vi "Serial.FrameCapture.vi"(7 "Over Time(mS)":u32=3000, 8 "error in (no error)":errorcluster caption="错误输入（无错误）", 9 "Input Text":string, 10 "baud rate (9600)":u32=9600 caption="BateRate(9600)", 11 "Serial":refnum<visa-resource-name>) -> (0 "error out":errorcluster caption="错误输出", 1 "Capture Text":string, 3 "Find?":bool)   [LabVIEW 2012, in "Lib_UEL.ATE.lvlib" / "Lib_2Voice.lvlib"]
uses:
  Lib_2Voice.lvlib
  <vilib>/Instr/_visa.llb/VISA Configure Serial Port (Instr).vi
panel:
  out "替换后偏移量":i32
  out "Time Count":u32
  in  "停止":bool
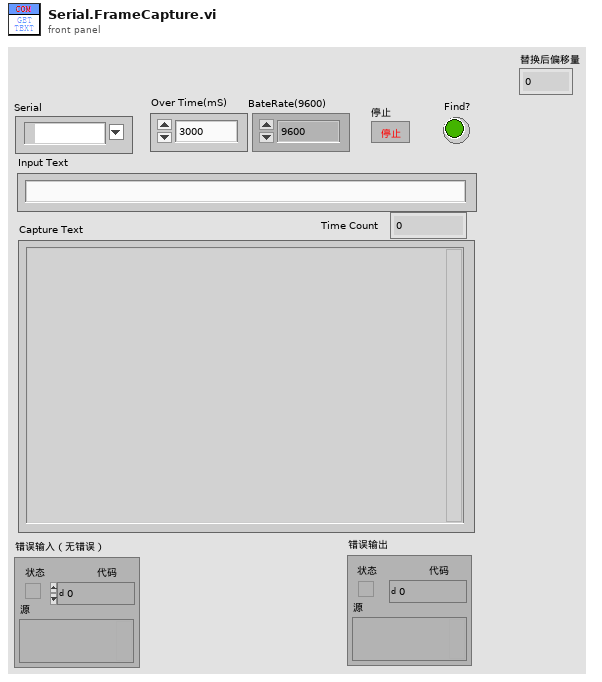
[diagram p1: front panel]
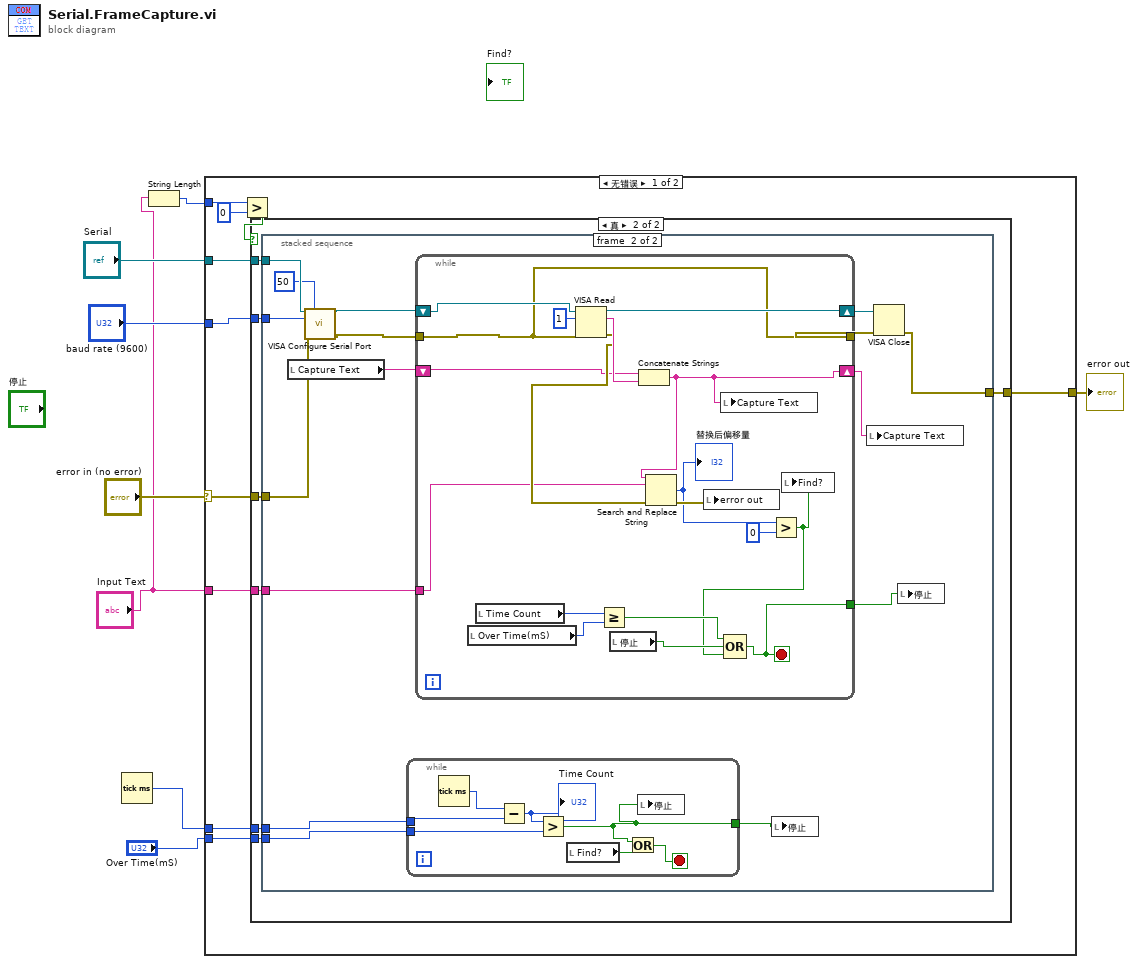
[diagram p0: block diagram]
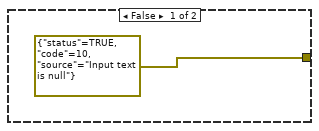
[diagram p2: hidden frame]
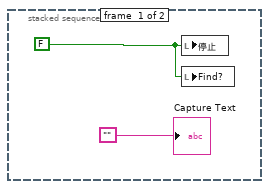
[diagram p3: hidden frame]
diagram:
  n1 = Tick Count (ms)() -> (millisecond timer value=w4:u32)
  n2 = String Length(string="Input Text") -> (length=w2:i32)
  n3 = case shown="无错误" "error in (no error)" {
    selector: "error in (no error)" -> [w17 w70]
    tunnel: "baud rate (9600)" -> [w18 _]
    tunnel: [w13 w70] -> w7
    tunnel: "Serial" -> [w16 _]
    tunnel: w4 -> [w15 _]
    tunnel: "Over Time(mS)" -> [w14 _]
    tunnel: "Input Text" -> [w12 _]
    tunnel: w2 -> [w11 _]
    frame No Error {
      n4 = Greater?(x=w11, y=0) -> (0:w9:bool)
      n5 = case shown="真" w9 {
        tunnel: w18 -> [_ w26]
        tunnel: w17 -> [_ w25]
        tunnel: w16 -> [_ w24]
        tunnel: w15 -> [_ w23]
        tunnel: w14 -> [_ w22]
        tunnel: [errorcluster {"status"=TRUE, "code"=10, "source"="Input text is null"} ("error out") w21] -> w13
        tunnel: w12 -> [_ w20]
        frame False {
        }
        frame True {
          n6 = stacked-sequence {
            tunnel: w26 -> [_ w44]
            tunnel: w25 -> [_ w43]
            tunnel: w24 -> [_ w42]
            tunnel: w23 -> [_ w40]
            tunnel: w22 -> [_ w39]
            tunnel: [_ w36] -> w21
            tunnel: w20 -> [_ w34]
            frame #0 {
              w28 = FALSE ("停止")
              n7 = local write "停止"(w28) -> ()
              n8 = local write "Find?"(w28) -> ()
              "Capture Text" <- ""
            }
            frame #1 {
              n9 = local read "Capture Text"() -> (w32:string)
              n10 = call-poly "VISA Configure Serial Port"("VISA resource name"=w42, "timeout (10sec)"=u32 50, "baud rate (9600)"=w44, "error in (no error)"=w43) -> ("VISA resource name out"=w30:refnum<visa-resource-name>, "error out"=w29:errorcluster)  [unwired: 10 in]
              n11 = while {
                tunnel: w40 -> [w50]
                tunnel: w39 -> [w48]
                tunnel: [w45] -> w35
                stop <- w47 stop-if-true
                n12 = Tick Count (ms)() -> (millisecond timer value=w51:u32)
                n13 = Subtract(x=w51, y=w50) -> (x-y=w49:u32)
                "Time Count" <- w49
                n14 = Greater?(x=w49, y=w48) -> (0:w45:bool)
                n15 = local read "Find?"() -> (w46:bool)
                n16 = Or(x=w45, y=w46) -> (x .or. y?=w47:bool)
                n17 = local write "停止"(w45) -> ()
              }
              n18 = while {
                shift-right: [w69] -> w38
                shift-left: w30 -> [w53]
                tunnel: w29 -> [w52]
                tunnel: [w52] -> w37
                tunnel: w34 -> [w60]
                tunnel: [w59] -> w33
                shift-right: [w55] -> w31
                shift-left: w32 -> [w56]
                stop <- w59 stop-if-true
                n19 = local read "Over Time(mS)"() -> (w64:u32)
                n20 = local read "Time Count"() -> (w65:u32)
                n21 = VISA Read(VISA resource name=w53, byte count=u32 1 ("字节总数"), error in (no error)=w52) -> (VISA resource name out=w69:refnum<visa-resource-name>, read buffer=w67:string, error out=w61:errorcluster)  [unwired: 1 out]
                n22 = Greater Or Equal?(x=w65, y=w64) -> (x >= y?=w63:bool)
                n23 = local read "停止"() -> (w66:bool)
                n24 = Concatenate Strings(w56, w67) -> (w55:string)
                n25 = Search and Replace String(input string=w55, search string=w60, error in=w61) -> (number of replacements=w54:i32, error out=w57:errorcluster)  [unwired: 5 in, 2 out]
                "替换后偏移量" <- w54
                n26 = local write "error out"(w57) -> ()
                n27 = local write "Capture Text"(w55) -> ()
                n28 = Greater?(x=w54, y=0) -> (0:w58:bool)
                n29 = Compound Arithmetic op=OR(w63, w66, w58) -> (w59:bool)
                n30 = local write "Find?"(w58) -> ()
              }
              n31 = local write "停止"(w35) -> ()
              n32 = local write "Capture Text"(w31) -> ()
              n33 = VISA Close(VISA resource name=w38, error in (no error)=w37) -> (error out=w36:errorcluster)
              n34 = local write "停止"(w33) -> ()
            }
          }
        }
      }
    }
    frame Error {
    }
  }
  "error out" <- w7
